vi "WPI_DMARepackSample.vi"(10 "Data":u32[](array[numeric])) -> (1 "Overun":bool, 2 "String Out":string)   [LabVIEW 2017]
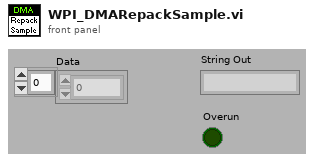
[diagram p1: front panel]
types:
  T1 = typedef "WPI_DMAChannelTypeEnum.ctl" = enum16{"AI (Raw)", "AI (Avg)", "Accumulator", "DI (Raw) Onboard", "DI (Filtered) Onboard", "DI (Raw) MXP", "DI (Filtered) MXP", "Analog Trigger", "Counter", "Counter (Timer)", "Encoder", "Encoder (Timer)", "Time Stamp"}
  T2 = cluster{"Channel Type":T1, "Channel Number":u8}[]
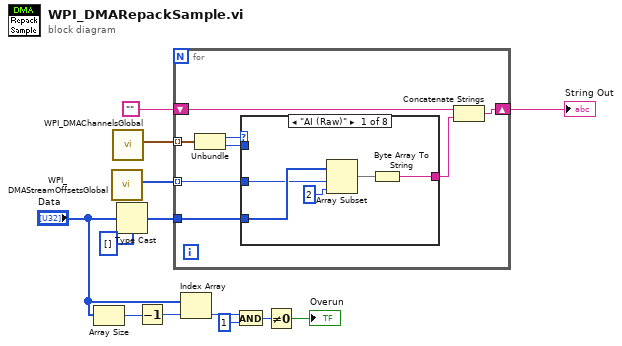
[diagram p0: block diagram]
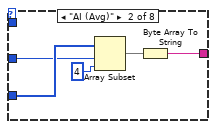
[diagram p2: hidden frame]
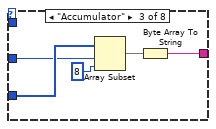
[diagram p3: hidden frame]
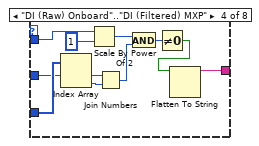
[diagram p4: hidden frame]
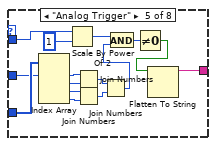
[diagram p5: hidden frame]
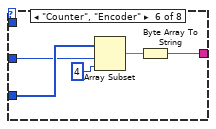
[diagram p6: hidden frame]
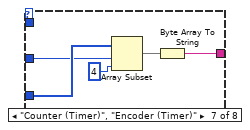
[diagram p7: hidden frame]
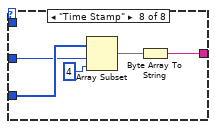
[diagram p8: hidden frame]
diagram:
  n1 = Array Size(array="Data") -> (size(s)=w9:i32)
  n2 = call <vilib>:"WPI_DMAStreamOffsetsGlobal.vi"() -> ("StreamOffsets"=w12:i32[])  [unwired: 3 in, 8 out]
  n3 = call <vilib>:"WPI_DMAChannelsGlobal.vi"() -> ("Channels Out"=w13:T2)  [unwired: 4 in, 7 out]
  n4 = Type Cast(type=u8[] [] ("Data"), x="Data") -> (*(type *) &x=w2:u8[])
  n5 = Decrement(x=w9) -> (x-1=w8:i32)
  n6 = for {
    tunnel: w13 -> [w21] mode=indexing
    tunnel: w12 -> [w19] mode=indexing
    tunnel: w2 -> [w18]
    shift-right: [w17] -> w10
    shift-left: "" -> [w16]
    n7 = Unbundle(w21) -> ("Channel Type"=w20:T1, "Channel Number"=w14:u8)
    n8 = case shown="\"AI (Raw)\"" w20 {
      tunnel: w19 -> [w25 w30 w35 w46 w61 w66 w71 w76]
      tunnel: w18 -> [w26 w31 w36 w47 w62 w67 w72 w77]
      tunnel: [w22 w27 w32 w38 w56 w63 w68 w73] -> w15
      tunnel: w14 -> [_ _ _ w42 w59 _ _ _]
      frame "AI (Raw)" {
        n9 = Array Subset(array=w26, index=w25, length=2) -> (w23:u8[])
        n10 = Byte Array To String(unsigned byte array=w23) -> (string=w22:string)
      }
      frame "AI (Avg)" {
        n11 = Array Subset(array=w31, index=w30, length=4) -> (w28:u8[])
        n12 = Byte Array To String(unsigned byte array=w28) -> (string=w27:string)
      }
      frame "Accumulator" {
        n13 = Array Subset(array=w36, index=w35, length=8) -> (w33:u8[])
        n14 = Byte Array To String(unsigned byte array=w33) -> (string=w32:string)
      }
      frame "DI (Raw) Onboard".."DI (Filtered) MXP" {
        n15 = Index Array(array=w47, index #1=w46) -> (element #1=w44:u8, element #2=w45:u8)  [unwired: 1 in]
        n16 = Scale By Power Of 2(n=w42, x=u16 1) -> (x*2^n=w40:u16)
        n17 = Join Numbers(hi=w44, lo=w45) -> ((hi.lo)=w41:u16)
        n18 = And(x=w40, y=w41) -> (x .and. y?=w39:u16)
        n19 = Not Equal To 0?(x=w39) -> (x != 0?=w37:bool)
        n20 = Flatten To String(anything=w37) -> (data string=w38:string)  [unwired: 1 in, 4 out]
      }
      frame "Analog Trigger" {
        n21 = Index Array(array=w62, index #1=w61) -> (element #1=w53:u8, element #2=w52:u8, element #3=w51:u8, element #4=w50:u8)  [unwired: 3 in]
        n22 = Scale By Power Of 2(n=w59, x=u32 1) -> (x*2^n=w58:u32)
        n23 = Join Numbers(hi=w53, lo=w52) -> ((hi.lo)=w49:u16)
        n24 = Join Numbers(hi=w51, lo=w50) -> ((hi.lo)=w48:u16)
        n25 = Join Numbers(hi=w49, lo=w48) -> ((hi.lo)=w54:u32)
        n26 = And(x=w58, y=w54) -> (x .and. y?=w57:u32)
        n27 = Not Equal To 0?(x=w57) -> (x != 0?=w55:bool)
        n28 = Flatten To String(anything=w55) -> (data string=w56:string)  [unwired: 1 in, 4 out]
      }
      frame "Counter", "Encoder" {
        n29 = Array Subset(array=w67, index=w66, length=4) -> (w64:u8[])
        n30 = Byte Array To String(unsigned byte array=w64) -> (string=w63:string)
      }
      frame "Counter (Timer)", "Encoder (Timer)" {
        n31 = Array Subset(array=w72, index=w71, length=4) -> (w69:u8[])
        n32 = Byte Array To String(unsigned byte array=w69) -> (string=w68:string)
      }
      frame "Time Stamp" {
        n33 = Array Subset(array=w77, index=w76, length=4) -> (w74:u8[])
        n34 = Byte Array To String(unsigned byte array=w74) -> (string=w73:string)
      }
    }
    n35 = Concatenate Strings(w16, w15) -> (w17:string)
  }
  "String Out" <- w10
  n36 = Index Array(array="Data", index=w8) -> (element=w7:u32)
  n37 = And(x=w7, y=u32 1) -> (x .and. y?=w5:u32)
  n38 = Not Equal To 0?(x=w5) -> (x != 0?=→"Overun":bool)
